vi "Lectura del  Graficador.vi"() -> ()   [LabVIEW 2020]
panel:
  out "Limite":dbl
  out "Temp":dbl
  out "Alarma":bool
  in  "stop":bool
  out "Datos Recolectados":dynamicdata(graph)
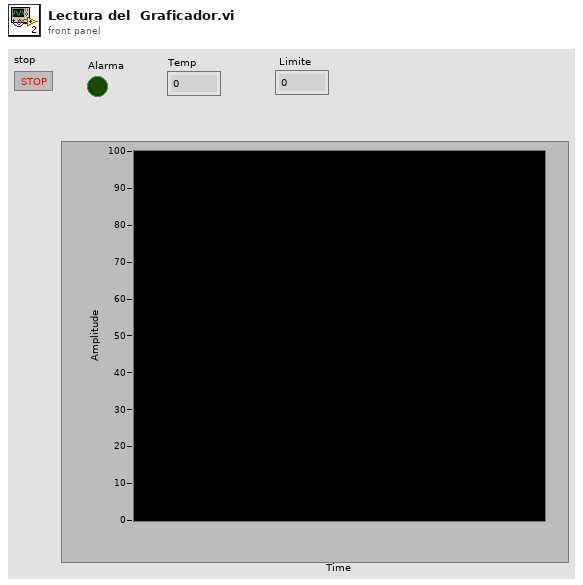
[diagram p1: front panel]
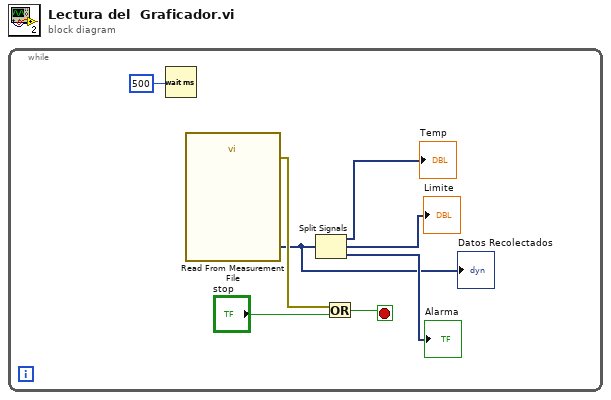
[diagram p0: block diagram]
diagram:
  n1 = while {
    stop <- w6 stop-if-true
    n2 = Wait (ms)(milliseconds to wait=500) -> ()  [unwired: 1 out]
    n3 = call "Read From Measurement File"() -> ("error out"=w7:errorcluster, "Signals"=w2:dynamicdata)  [unwired: 6 in, 4 out]
    "Datos Recolectados" <- w2
    n4 = Split Signals(w2) -> (→"Temp":dynamicdata, →"Limite":dynamicdata, →"Alarma":dynamicdata)  [unwired: 3 in]
    n5 = Or(x=w7, y="stop") -> (x .or. y?=w6:bool)
  }
